vi "Convert Buffer.vi"(1 "Buffer":string) -> (0 "Out String":string)   [LabVIEW 2019]
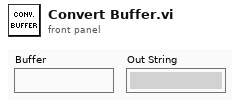
[diagram p1: front panel]
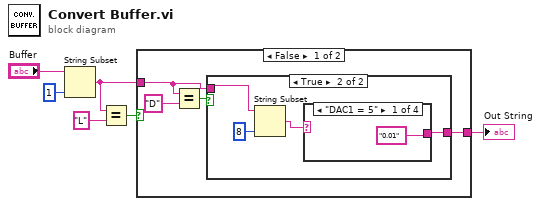
[diagram p0: block diagram]
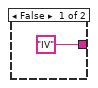
[diagram p2: hidden frame]
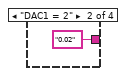
[diagram p3: hidden frame]
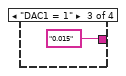
[diagram p4: hidden frame]
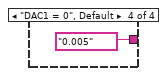
[diagram p5: hidden frame]
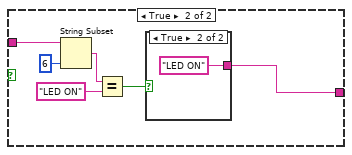
[diagram p6: hidden frame]
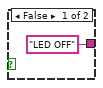
[diagram p7: hidden frame]
diagram:
  n1 = String Subset(string="Buffer", length (rest)=1 ("length (rest)")) -> (substring=w3:string)  [unwired: 1 in]
  n2 = Equal?(x=w3, y="L") -> (x = y?=w4:bool)
  n3 = case shown="False" w4 {
    tunnel: w3 -> [w7 w23]
    tunnel: [w8 w20] -> w2
    frame False {
      n4 = Equal?(x=w7, y="D") -> (x = y?=w9:bool)
      n5 = case shown="True" w9 {
        tunnel: ["IV" ("y") w13] -> w8
        tunnel: w7 -> [_ w14]
        frame False {
        }
        frame True {
          n6 = String Subset(string=w14, length (rest)=8 ("length (rest)")) -> (substring=w12:string)  [unwired: 1 in]
          n7 = case shown="\"DAC1 = 5\"" w12 {
            tunnel: ["0.01" ("y") "0.02" ("y") "0.015" ("y") "0.005" ("y")] -> w13
            frame "DAC1 = 5" {
            }
            frame "DAC1 = 2" {
            }
            frame "DAC1 = 1" {
            }
            frame "DAC1 = 0", Default {
            }
          }
        }
      }
    }
    frame True {
      n8 = String Subset(string=w23, length (rest)=6 ("length (rest)")) -> (substring=w25:string)  [unwired: 1 in]
      n9 = Equal?(x=w25, y="LED ON") -> (x = y?=w22:bool)
      n10 = case shown="True" w22 {
        tunnel: ["LED OFF" ("y") "LED ON" ("y")] -> w20
        frame False {
        }
        frame True {
        }
      }
    }
  }
  "Out String" <- w2
